vi "LL Offsets.vi"() -> ()   [LabVIEW 2019]
panel:
  in  "LL Y Offset":dbl
  in  "LL X Offset":dbl
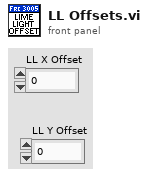
[diagram p1: front panel]
diagram:
